vi "PCAN_Terminal.vi"() -> ()   [LabVIEW 2010]
panel:
  out "Version":string
  in  "type":i32(ring) items=["standart", "extended"]
  in  "baud":u16(ring)=20 items=["1M"=20, "500K"=28, "250K"=284, "125K"=796, "100K"=17199, "50K"=18223, "20K"=21295, "10K"=26415, "5K"=32639]
  in  "TPCANMsg To Write":T1 {"ID" format="%x"; "MSGTYPE" items=["STATUS"=128, "EXTENDED"=2, "RTR"=1, "DATA MSG"=0]; "aDATA" format="%x"}
  in  "Write":bool
  out "Last Error":string
  out "TPCANMsg":T1 {"ID" format="%x"; "MSGTYPE" items=["STATUS"=128, "EXTENDED"=2, "RTR"=1, "DATA MSG"=0]; "aDATA" format="%x"}
  in  "stop":bool
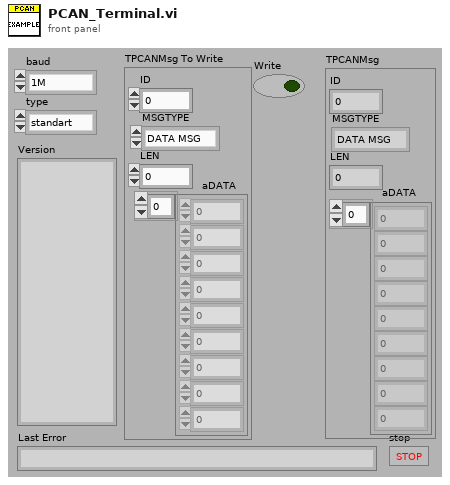
[diagram p1: front panel]
types:
  T1 = cluster{"ID":u32, "MSGTYPE":u8, "LEN":u8, "aDATA":u8[]}
  T2 = cluster{"Is Warning":bool, "Is Error":bool, "Message":string}
  T3 = typedef "PCAN_ERROR.ctl" = i32
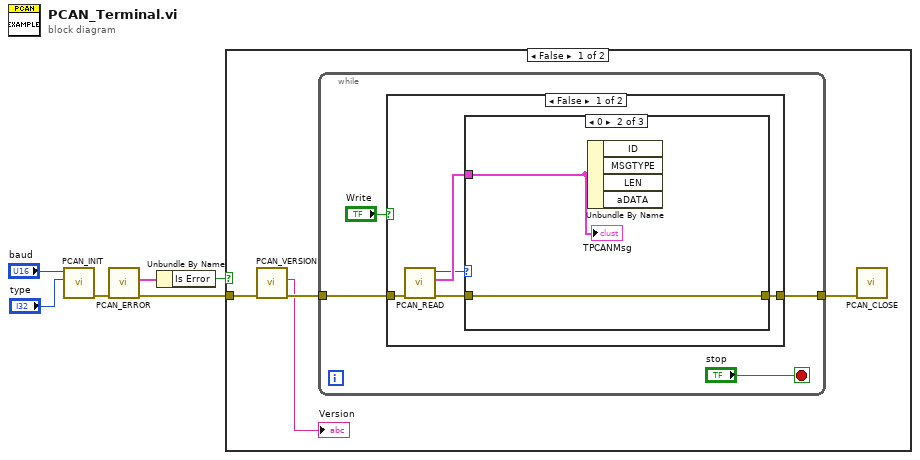
[diagram p0: block diagram]
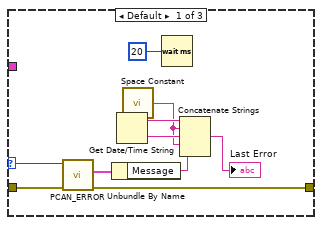
[diagram p2: hidden frame]
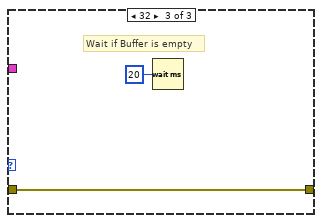
[diagram p3: hidden frame]
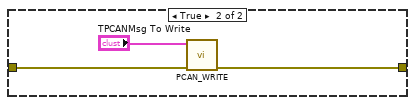
[diagram p4: hidden frame]
diagram:
  n1 = call "PCAN_INIT.vi"("Msg Type"="type", "BTR0BTR1"="baud") -> ("error out"=w4:errorcluster)  [unwired: 2 in, 7 out]
  n2 = call "PCAN_ERROR.vi"("error in (no error)"=w4) -> ("error out"=w3:errorcluster, "PCAN error"=w2:T2)  [unwired: 1 in, 8 out]
  n3 = Unbundle By Name(w2) -> ("Is Error"=w1:bool)
  n4 = case shown="False" w1 {
    tunnel: w3 -> [w7 _]
    frame False {
      n5 = call "PCAN_VERSION.vi"("error in (no error)"=w7) -> ("error out"=w9:errorcluster, "lpszTextBuff"=→"Version":string)  [unwired: 1 in, 8 out]
      n6 = while {
        tunnel: w9 -> [w14]
        tunnel: [w13] -> w10
        stop <- "stop" stop-if-true
        n7 = case shown="False" "Write" {
          tunnel: w14 -> [w19 w36]
          tunnel: [w15 w35] -> w13
          frame False {
            n8 = call "PCAN_READ.vi"("error in (no error)"=w19) -> ("error out"=w16:errorcluster, "TPCANMsg"=w18:T1, "error"=w17:T3)  [unwired: 1 in, 7 out]
            n9 = case shown="0" w17 {
              selector: w17 -> [w28 _ _]
              tunnel: w18 -> [_ w30 _]
              tunnel: w16 -> [w29 w31 w32]
              tunnel: [w27 w31 w32] -> w15
              frame Default {
                n10 = call "PCAN_ERROR.vi"("error in (no error)"=w29, "Error Code"=w28) -> ("error out"=w27:errorcluster, "PCAN error"=w26:T2)  [unwired: 8 out]
                n11 = Unbundle By Name(w26) -> ("Message"=w21:string)
                n12 = Get Date/Time String() -> (date string=w24:string, time string=w23:string)  [unwired: 3 out]
                n13 = call <vilib>:"Space Constant.vi"() -> ("String"=w20:string)
                n14 = Wait (ms)(milliseconds to wait=u32 20) -> ()  [unwired: 1 out]
                n15 = Concatenate Strings(w24, w20, w23, w20, w21) -> (→"Last Error":string)
              }
              frame 0 {
                n16 = Unbundle By Name(w30) -> ()  [unwired: 4 out]
                "TPCANMsg" <- w30
              }
              frame 32 {
                # "Wait if Buffer is empty"
                n17 = Wait (ms)(milliseconds to wait=u32 20) -> ()  [unwired: 1 out]
              }
            }
          }
          frame True {
            n18 = call "PCAN_WRITE.vi"("error in (no error)"=w36, "TPCANMsg"="TPCANMsg To Write") -> ("error out"=w35:errorcluster)  [unwired: 1 in, 8 out]
          }
        }
      }
      n19 = call "PCAN_CLOSE.vi"("error in (no error)"=w10) -> ()  [unwired: 11 out]
    }
    frame True {
    }
  }
